vi "IR PAIR INTERFACE USIND DAQ CARD.vi"() -> ()   [LabVIEW 2021]
uses:
  <vilib>/DAQmx/read.llb/DAQmx Read (Analog DBL 1Chan 1Samp).vi
  <vilib>/DAQmx/create/channels.llb/DAQmx Create Channel (AI-Voltage-Basic).vi
  <vilib>/DAQmx/miscellaneous.llb/DAQmx Fill In Error Info.vi
panel:
  out "Meter":dbl(knob) scale=0.0..10.0
  in  "STOP":bool
  out "OBJECT DETECTION INDICATOR":bool
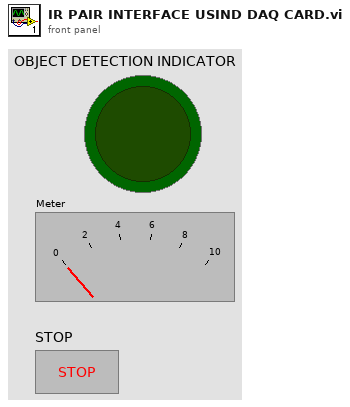
[diagram p1: front panel]
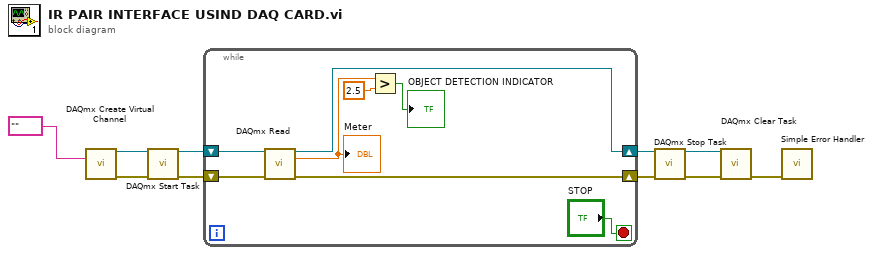
[diagram p0: block diagram]
diagram:
  n1 = call-poly <vilib>:"DAQmx Create Virtual Channel.vi"("physical channels"=tag "") -> ("task out"=w4:refnum<k21>, "error out"=w3:errorcluster)  [unwired: 13 in]
  n2 = call <vilib>:"DAQmx Start Task.vi"("task/channels in"=w4, "error in"=w3) -> ("task out"=w2:refnum<k21>, "error out"=w1:errorcluster)  [unwired: 12 in]
  n3 = while {
    shift-right: [w16] -> w10
    shift-left: w2 -> [w18]
    shift-right: [w15] -> w9
    shift-left: w1 -> [w17]
    stop <- "STOP" stop-if-true
    n4 = call-poly <vilib>:"DAQmx Read.vi"("task/channels in"=w18, "error in"=w17) -> ("task out"=w16:refnum<k21>, "data"=w11:dbl, "error out"=w15:errorcluster)  [unwired: 11 in]
    "Meter" <- w11
    n5 = Greater?(x=w11, y=2.5) -> (0:→"OBJECT DETECTION INDICATOR":bool)
  }
  n6 = call <vilib>:"DAQmx Stop Task.vi"("task/channels in"=w10, "error in"=w9) -> ("task out"=w8:refnum<k21>, "error out"=w7:errorcluster)  [unwired: 12 in]
  n7 = call <vilib>:"DAQmx Clear Task.vi"("task in"=w8, "error in"=w7) -> ("error out"=w6:errorcluster)  [unwired: 13 in]
  n8 = call <vilib>:"Simple Error Handler.vi"("error in (no error)"=w6) -> ()  [unwired: 4 in, 5 out]
